vi "Start.vi"(0 "object in":refnum<class "DAQ.lvclass">, 5 "error in (no error)":errorcluster) -> (14 "object out":refnum<class "DAQ.lvclass">, 19 "error out":errorcluster)   [LabVIEW 2021, in "DAQ.lvclass"]
uses:
  DAQ.lvclass
  DAQ.lvclass/DAQ.ctl
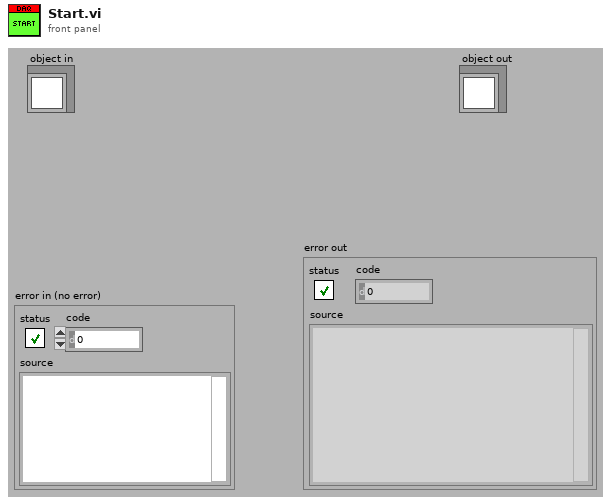
[diagram p1: front panel]
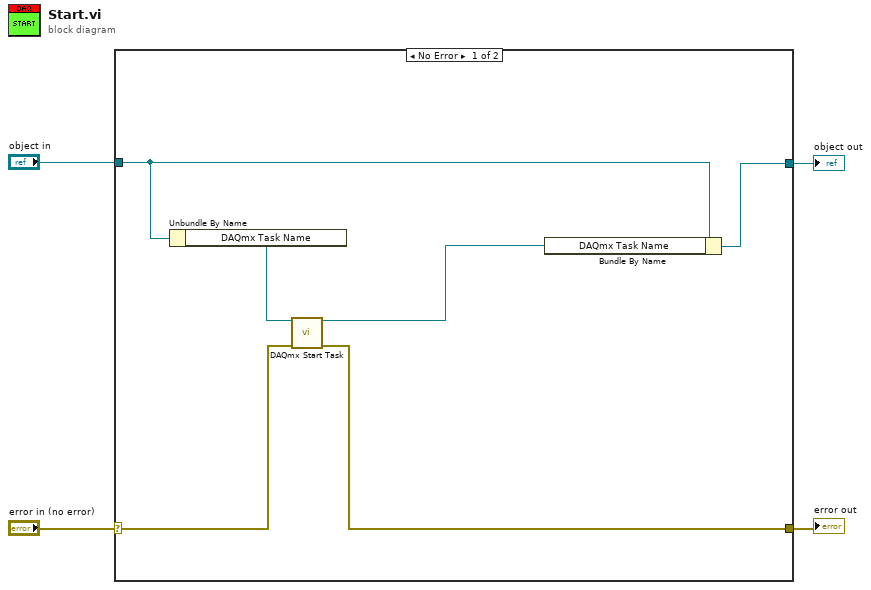
[diagram p0: block diagram]
diagram:
  n1 = case shown="No Error" "error in (no error)" {
    selector: "error in (no error)" -> [w9 w12]
    tunnel: [w5 w12] -> w3
    tunnel: [w7 w11] -> w1
    tunnel: "object in" -> [w8 w11]
    frame No Error {
      n2 = Unbundle By Name(w8) -> ("DAQmx Task Name"=w10:refnum<k21>)
      n3 = call <vilib>:"DAQmx Start Task.vi"("task/channels in"=w10, "error in"=w9) -> ("task out"=w6:refnum<k21>, "error out"=w5:errorcluster)  [unwired: 12 in]
      n4 = Bundle By Name(cluster=w8, "DAQmx Task Name"=w6) -> (w7:refnum<class "DAQ.lvclass">)
    }
    frame Error {
    }
  }
  "error out" <- w3
  "object out" <- w1
